vi "ReadExEventInterrupts.vi"() -> ()   [LabVIEW 2015]
uses:
  GPS_Driver_Global.vi
panel:
  in  "Path to FITS Header File":path=path "C:/Users/Public/Documents/SI Image SGL II -/Other Parameters.txt"
  out "# Entries After":i16
  in  "# Entries Before":i16
  out "Close Min":u32
  out "Close Maj":u32
  out "Open Min":u32
  out "Open Maj":u32
  out "error out":errorcluster
  in  "error in (no error)":errorcluster
  # "Major UNIX Time:"
  # "Minor UNIX Time:"
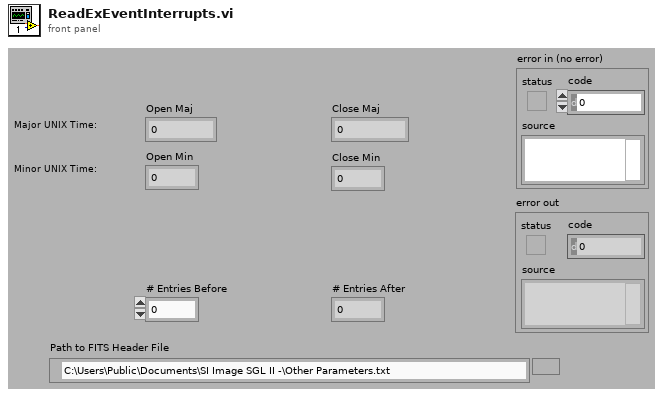
[diagram p1: front panel]
types:
  T1 = cluster{"Close":cluster{"Time":string, "Error":string}, "Open":cluster{"Time":string, "Error":string}, "Date":cluster{"Date":string, "Error":string}}
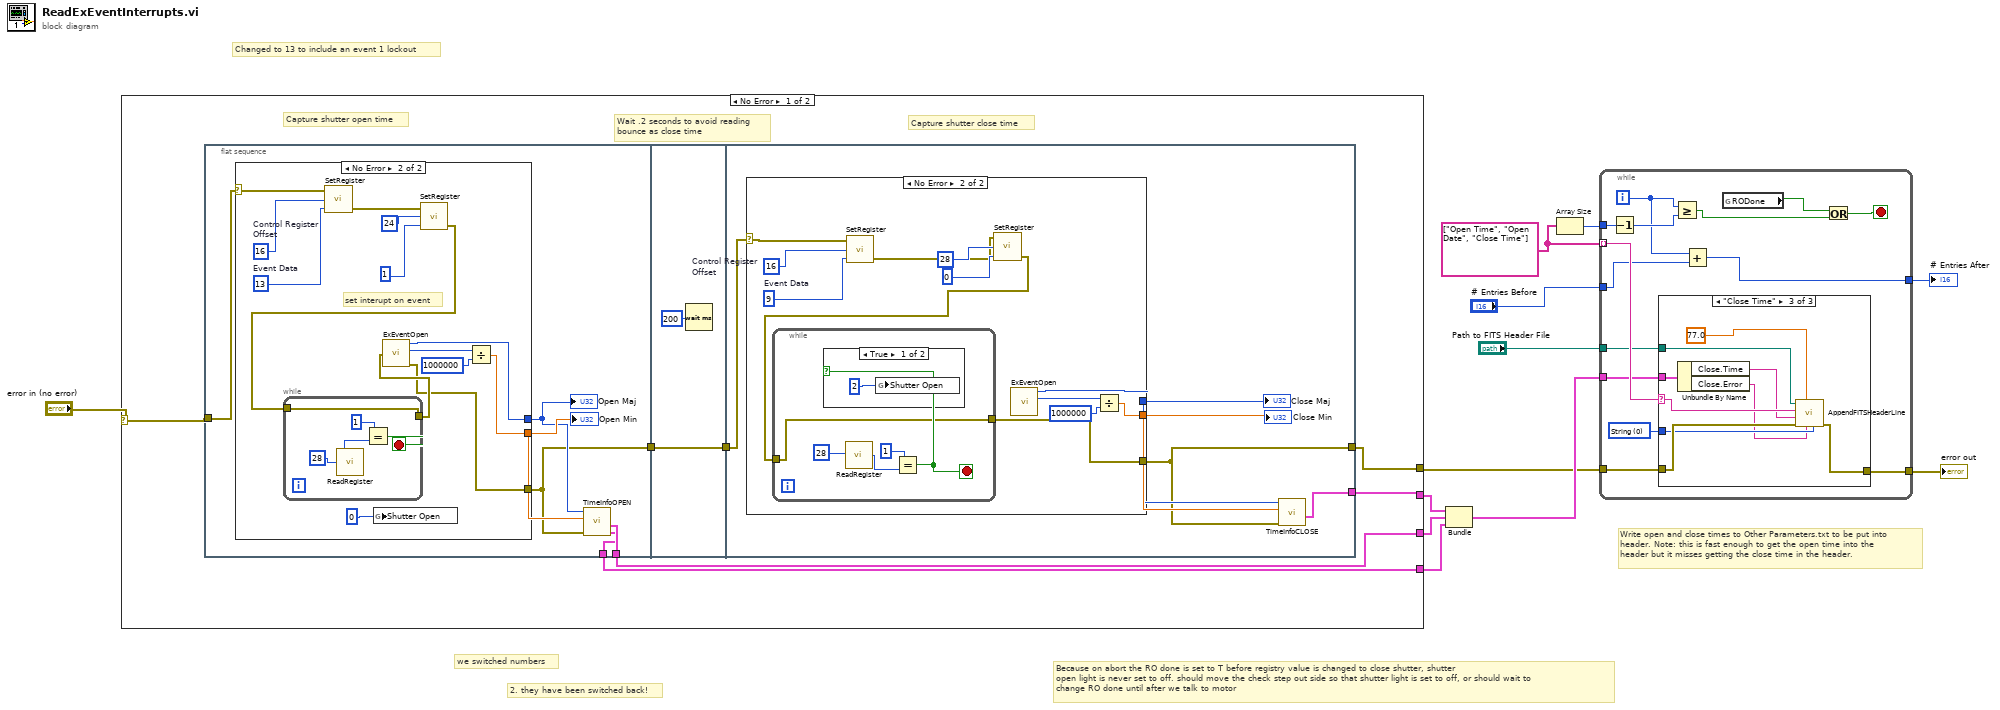
[diagram p0: block diagram]
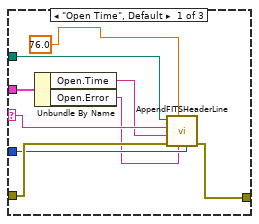
[diagram p2: hidden frame]
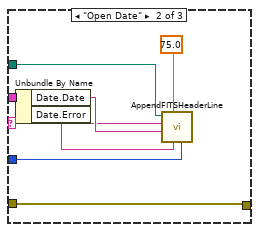
[diagram p3: hidden frame]
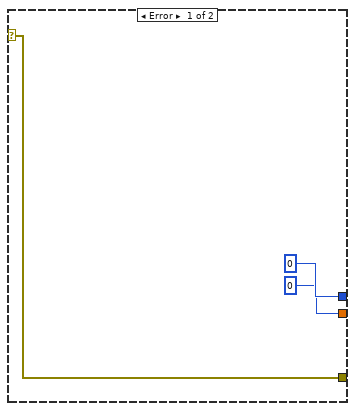
[diagram p4: hidden frame]
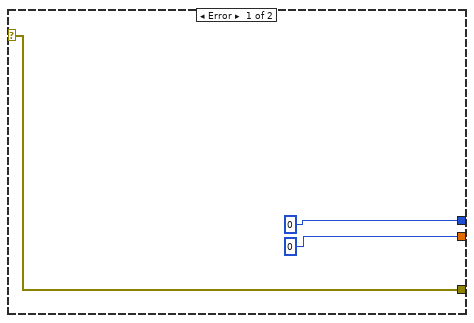
[diagram p5: hidden frame]
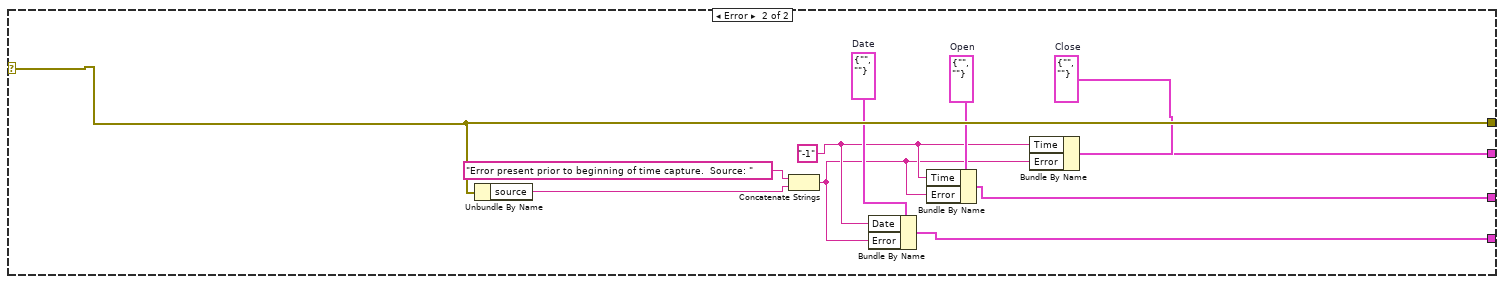
[diagram p7: hidden frame]
diagram:
  w12 = string[] ["Open Time", "Open Date", "Close Time"]
  # "Changed to 13 to include an event 1 lockout"
  # "Because on abort the RO done is set to T before registry value is changed to close shutter, shutter\nopen light is never set to off. should move the check step out side so that shutter light is set to off, or should wait to \nchange RO done until after we talk to motor"
  # "2. they have been switched back!"
  # "we switched numbers"
  # "Write open and close times to Other Parameters.txt to be put into\nheader. Note: this is fast enough to get the open time into the \nheader but it misses getting the close time in the header."
  n1 = case shown="No Error" "error in (no error)" {
    selector: "error in (no error)" -> [w14 w86]
    tunnel: [w13 w86] -> w7
    tunnel: [w19 w79] -> w8
    tunnel: [w18 w82] -> w9
    tunnel: [w15 w80] -> w1
    frame No Error {
      # "Capture shutter close time"
      # "Wait .2 seconds to avoid reading \nbounce as close time"
      # "Capture shutter open time"
      n2 = flat-sequence {
        tunnel: w14 -> [w23]
        tunnel: [w22] -> w19
        tunnel: [w21] -> w16
        tunnel: [w20] -> w15
        tunnel: [w48] -> w17
        tunnel: w16 -> [w48]
        tunnel: [w52] -> w18
        tunnel: w17 -> [w51]
        tunnel: [w50] -> w13
        frame #0 {
          n3 = case shown="No Error" w23 {
            selector: w23 -> [w26 w38]
            tunnel: [0 w34] -> w25
            tunnel: [w26 w36] -> w21
            tunnel: [0 w35] -> w24
            frame Error {
            }
            frame No Error {
              w41 = 13  # Event Data
              w42 = 16  # Control Register Offset
              # "set interupt on event"
              n4 = call "SetRegister.vi"("Data"=w41, "Offset"=w42, "error in (no error)"=w38) -> ("error out"=w31:errorcluster)  [unwired: 2 in]
              n5 = global write "GPS_Driver_Global.vi" "Shutter Open"(0) -> ()
              n6 = call "SetRegister.vi"("Data"=1, "Offset"=24, "error in (no error)"=w31) -> ("error out"=w30:errorcluster)  [unwired: 2 in]
              n7 = while {
                tunnel: w30 -> [w44]
                tunnel: [w44] -> w37
                stop <- w45 stop-if-true
                n8 = call "ReadRegister.vi"("Offset"=28) -> ("Return"=w47:i32)  [unwired: 3 in, 1 out]
                n9 = Equal?(x=1, y=w47) -> (x = y?=w45:bool)
              }
              n10 = call "ExEventOpen.vi"("error in (no error)"=w37) -> ("Major Time"=w35:u32, "Minor Time"=w40:u32, "error out"=w36:errorcluster)  [unwired: 1 in]
              n11 = Divide(x=w40, y=1000000) -> (x/y=w34:dbl)
            }
          }
          "Open Min" <- w25
          "Open Maj" <- w24
          n12 = call "TimeInfoOPEN.vi"("error in (no error)"=w21, "Minor Time"=w25, "Major Time"=w24) -> ("Date"=w20:cluster{"Date":string, "Error":string}, "Open"=w22:cluster{"Time":string, "Error":string})  [unwired: 6 in]
        }
        frame #1 {
          n13 = Wait (ms)(milliseconds to wait=200) -> ()  [unwired: 1 out]
        }
        frame #2 {
          n14 = case shown="No Error" w51 {
            selector: w51 -> [w55 w65]
            tunnel: [0 w59] -> w54
            tunnel: [w55 w58] -> w50
            tunnel: [0 w60] -> w53
            frame Error {
            }
            frame No Error {
              w68 = 9  # Event Data
              w69 = 16  # Control Register Offset
              n15 = call "SetRegister.vi"("Data"=w68, "Offset"=w69, "error in (no error)"=w65) -> ("error out"=w61:errorcluster)  [unwired: 2 in]
              n16 = call "SetRegister.vi"("Data"=0 ("Event Data"), "Offset"=28 ("Control Register\nOffset"), "error in (no error)"=w61) -> ("error out"=w62:errorcluster)  [unwired: 2 in]
              n17 = while {
                tunnel: w62 -> [w71]
                tunnel: [w71] -> w58
                stop <- w73 stop-if-true
                n18 = call "ReadRegister.vi"("Offset"=28) -> ("Return"=w74:i32)  [unwired: 3 in, 1 out]
                n19 = Equal?(x=1, y=w74) -> (x = y?=w73:bool)
                n20 = case shown="True" w73 {
                  frame True {
                    n21 = global write "GPS_Driver_Global.vi" "Shutter Open"(2) -> ()
                  }
                  frame False {
                  }
                }
              }
              n22 = call "ExEventOpen.vi"() -> ("Major Time"=w60:u32, "Minor Time"=w67:u32)  [unwired: 2 in, 1 out]
              n23 = Divide(x=w67, y=1000000) -> (x/y=w59:dbl)
            }
          }
          "Close Maj" <- w53
          "Close Min" <- w54
          n24 = call "TimeInfoCLOSE.vi"("error in (no error)"=w50, "Minor Time"=w54, "Major Time"=w53) -> ("Close"=w52:cluster{"Time":string, "Error":string})  [unwired: 7 in]
        }
      }
    }
    frame Error {
      w78 = cluster{"Date":string, "Error":string} {"Date"="", "Error"=""}  # Date
      w83 = cluster{"Time":string, "Error":string} {"Time"="", "Error"=""}  # Close
      w81 = cluster{"Time":string, "Error":string} {"Time"="", "Error"=""}  # Open
      w77 = "-1"
      n25 = Unbundle By Name(w86) -> ("source"=w84:string)
      n26 = Concatenate Strings("Error present prior to beginning of time capture.  Source: ", w84) -> (w76:string)
      n27 = Bundle By Name(cluster=w78, "Date"=w77, "Error"=w76) -> (w80:cluster{"Date":string, "Error":string})
      n28 = Bundle By Name(cluster=w81, "Time"=w77, "Error"=w76) -> (w79:cluster{"Time":string, "Error":string})
      n29 = Bundle By Name(cluster=w83, "Time"=w77, "Error"=w76) -> (w82:cluster{"Time":string, "Error":string})
    }
  }
  n30 = Bundle("Close"=w9, "Open"=w8, "Date"=w1) -> (w11:T1)  [unwired: 1 in]
  n31 = Array Size(array=w12) -> (size(s)=w5:i32)
  n32 = while {
    tunnel: w7 -> [w100]
    tunnel: w12 -> [w98] mode=indexing
    tunnel: w5 -> [w97]
    tunnel: "# Entries Before" -> [w95]
    tunnel: w11 -> [w93]
    tunnel: "Path to FITS Header File" -> [w92]
    tunnel: [w91] -> w10
    tunnel: [w87] -> w3
    i -> [w94]
    stop <- w89 stop-if-true
    w96 = u16 0 items=["String", "Numeric", "Boolean"]
    n33 = Decrement(x=w97) -> (x-1=w99:i32)
    n34 = case shown="\"Close Time\"" w98 {
      selector: w98 -> [w107 w112 w125]
      tunnel: w100 -> [w109 w111 w126]
      tunnel: w96 -> [w108 w116 w124]
      tunnel: w93 -> [w104 w115 w121]
      tunnel: w92 -> [w106 w117 w122]
      tunnel: [w105 w111 w123] -> w91
      frame "Open Time", Default {
        n35 = Unbundle By Name(w104) -> ("Open.Time"=w103:string, "Open.Error"=w102:string)
        n36 = call "AppendFITSHeaderLine.vi"("Entry Type"=w108, "Comment"=w102, "Entry #"=76.0, "error in (no error)"=w109, "Element Value"=w103, "Element Name"=w107, "file path (dialog if empty)"=w106) -> ("error out"=w105:errorcluster)  [unwired: 3 in]
      }
      frame "Open Date" {
        n37 = Unbundle By Name(w115) -> ("Date.Date"=w114:string, "Date.Error"=w113:string)
        n38 = call "AppendFITSHeaderLine.vi"("Entry Type"=w116, "Comment"=w113, "Entry #"=75.0, "Element Value"=w114, "Element Name"=w112, "file path (dialog if empty)"=w117) -> ()  [unwired: 4 in, 1 out]
      }
      frame "Close Time" {
        n39 = Unbundle By Name(w121) -> ("Close.Time"=w120:string, "Close.Error"=w119:string)
        n40 = call "AppendFITSHeaderLine.vi"("Entry Type"=w124, "Comment"=w119, "Entry #"=77.0, "error in (no error)"=w126, "Element Value"=w120, "Element Name"=w125, "file path (dialog if empty)"=w122) -> ("error out"=w123:errorcluster)  [unwired: 3 in]
      }
    }
    n41 = Greater Or Equal?(x=w94, y=w99) -> (x >= y?=w90:bool)
    n42 = Add(x=w94, y=w95) -> (x+y=w87:i32)
    n43 = global read "GPS_Driver_Global.vi" "RODone"() -> (w88:bool)
    n44 = Or(x=w88, y=w90) -> (x .or. y?=w89:bool)
  }
  "error out" <- w10
  "# Entries After" <- w3
